vi "Do.vi"(8 "error in (no error)":errorcluster, 10 "Actor in":refnum<class "Actor.lvclass">, 11 "Ask Controller to Launch Results UI Msg":refnum<class "Ask Controller to Launch Results UI Msg.lvclass">) -> (0 "error out":errorcluster, 2 "Actor out":refnum<class "Actor.lvclass">)   [LabVIEW 2016, in "Controller UI.lvlib" / "Ask Controller to Launch Results UI Msg.lvclass"]
uses:
  <userlib>/Common Components/Controller UI/Messages/Ask Controller to Launch Results UI Msg/Ask Controller to Launch Results UI Msg.lvclass
  <vilib>/ActorFramework/Actor/Actor.lvclass
  <userlib>/Common Components/Controller UI/Controller UI.lvclass
  C:/Program Files (x86)/National Instruments/LabVIEW 2016/vi.lib/ActorFramework/Actor/Actor.lvclass
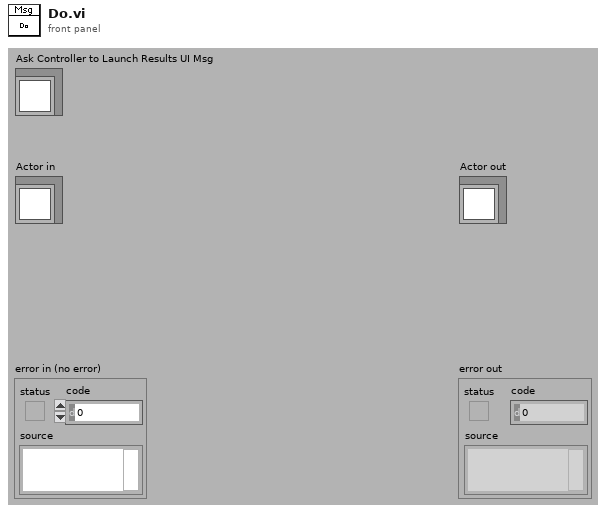
[diagram p1: front panel]
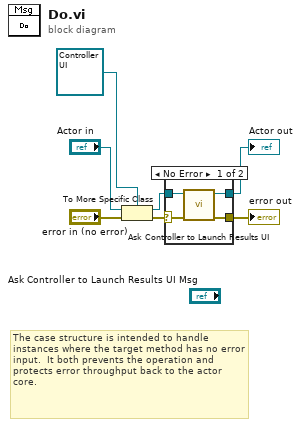
[diagram p0: block diagram]
diagram:
  # "The case structure is intended to handle instances where the target method has no error input.  It both prevents the operation and protects error throughput back to the actor core."
  n1 = To More Specific Class(target class=refnum<class "Controller UI.lvclass"> refnum ("Actor in"), reference="Actor in", error in="error in (no error)") -> (specific class reference=w7:refnum<class "Controller UI.lvclass">, error out=w3:errorcluster)
  n2 = case shown="No Error" w3 {
    selector: w3 -> [w8 w13]
    tunnel: w7 -> [w11 w12]
    tunnel: [w10 w13] -> w2
    tunnel: [w9 w12] -> w1
    frame No Error {
      n3 = call-dynamic "Ask Controller to Launch Results UI.vi"("error in (no error)"=w8, "Operator UI in"=w11) -> ("error out"=w10:errorcluster, "Operator UI out"=w9:refnum<class "Controller UI.lvclass">)  [unwired: 8 in]
    }
    frame Error {
    }
  }
  "error out" <- w2
  "Actor out" <- w1
